vi "Process.vi"(8 "error in (no error)":errorcluster, 10 "Initialize WDC in":refnum<class "Initialize WDC.lvclass">, 11 "Architecture.lvlib:Thread.lvclass":refnum<class "Thread.lvclass">) -> (0 "error out":errorcluster, 1 "Stop?":bool, 3 "Architecture.lvlib:Thread.lvclass 2":refnum<class "Thread.lvclass">)   [LabVIEW 2012, in "Wash Display Console.lvlib" / "Initialize WDC.lvclass"]
uses:
  Initialize WDC.lvclass
  Database/Database.lvclass
  Thread/Thread.lvclass
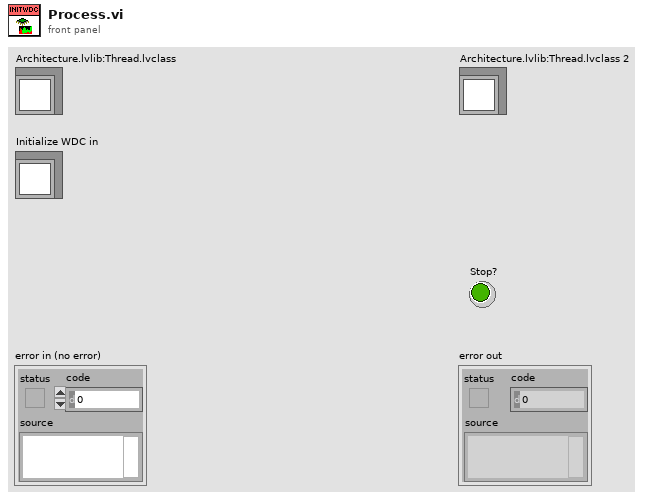
[diagram p1: front panel]
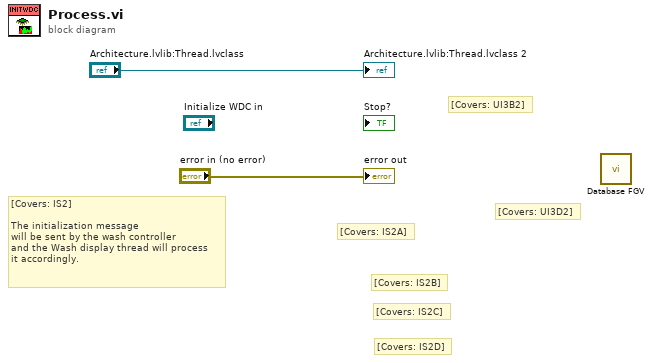
[diagram p0: block diagram]
diagram:
  # "[Covers: IS2D]"
  # "[Covers: IS2C]"
  # "[Covers: IS2B]"
  # "[Covers: IS2A]"
  # "[Covers: IS2]\n\nThe initialization message\nwill be sent by the wash controller\nand the Wash display thread will process\nit accordingly."
  # "[Covers: UI3D2]"
  # "[Covers: UI3B2]"
  n1 = call "Database FGV.vi"() -> ()  [unwired: 9 in, 3 out]
  "error out" <- "error in (no error)"
  "Architecture.lvlib:Thread.lvclass 2" <- "Architecture.lvlib:Thread.lvclass"
